vi "MainGUI.vi"(0 "reference in":refnum<class "UserManager.lvclass">, 5 "Error In":errorcluster) -> (14 "reference out":refnum<class "UserManager.lvclass">, 19 "Error Out":errorcluster)   [LabVIEW 2021]
doc: "This template is based off of the Queued Message Handler design pattern and the Queued Message Handler project template that ships with LabVIEW.\n\nThe main difference is that the queue is private to this module and communication between modules is performed via Broadcast and Request events.\n\nRequest events are wrapped in public API methods and are handled in the Event Handling Loop (EHL) of this VI. Any module can register for Broadcast events sent by this module. The EHL generates messages based on user interface actions.\n\nThe Message Handling Loop (MHL) processes messages generated by the EHL, or by other messages. The messages are string values, so new messages can be added easily to the Message Cases case structure in the MHL. Each message cluster can also provide an optional value for Message Data, which is a variant that can be converted to whatever message-specific data is required.\n_____\nBased on Delacor QMH Project Template 4.2.0.63.\n\n<b>Note:</b> This VI was modified by the <b>Validate DQMH Module</b> tool to have the module name be passed as the Additional Information parameter with an Error Reported broadcast.\n\n<b>Note:</b> This VI was modified by the <b>Validate DQMH Module</b> tool to call the Release Message Queue VI in the top-level Error case."
uses:
  .Externals/Library_TAF_UserManager/UserManager/UserManager/protected/UserManager_MessageData.ctl
  .Externals/Library_TAF_UserManager/UserManager/UserManager/UserManager.lvclass
panel:
  out "Last Command":string
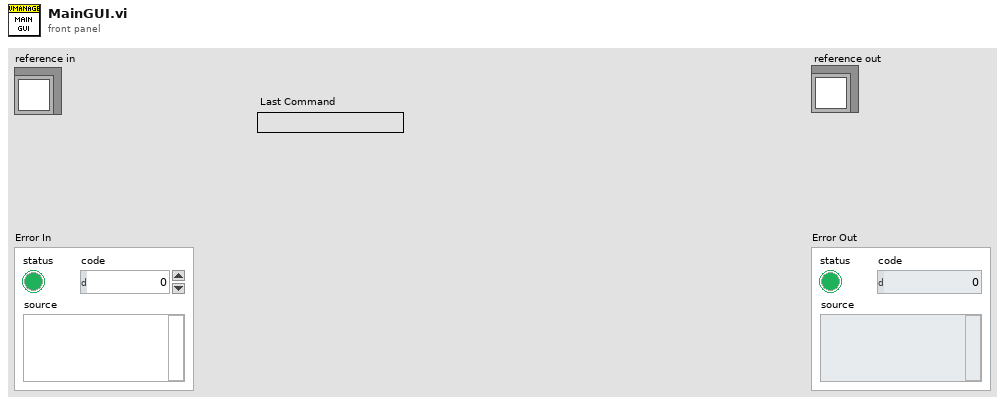
[diagram p1: front panel]
types:
  T1 = typedef "UserMananger.lvlib/UserManager.lvclass/UserManager_MessageData.ctl" = cluster{"ShowWindow":cluster{"Send":cluster{"Show":bool}, "Receive":cluster{"Dummy":bool}}}
  T2 = cluster{"Event":refnum<event-registration>, "Command":string, "MessageData":T1, "ReplyQueue":refnum<queue>}
  T3 = cluster{"ReplyQueue":refnum<queue>, "Data":variant}
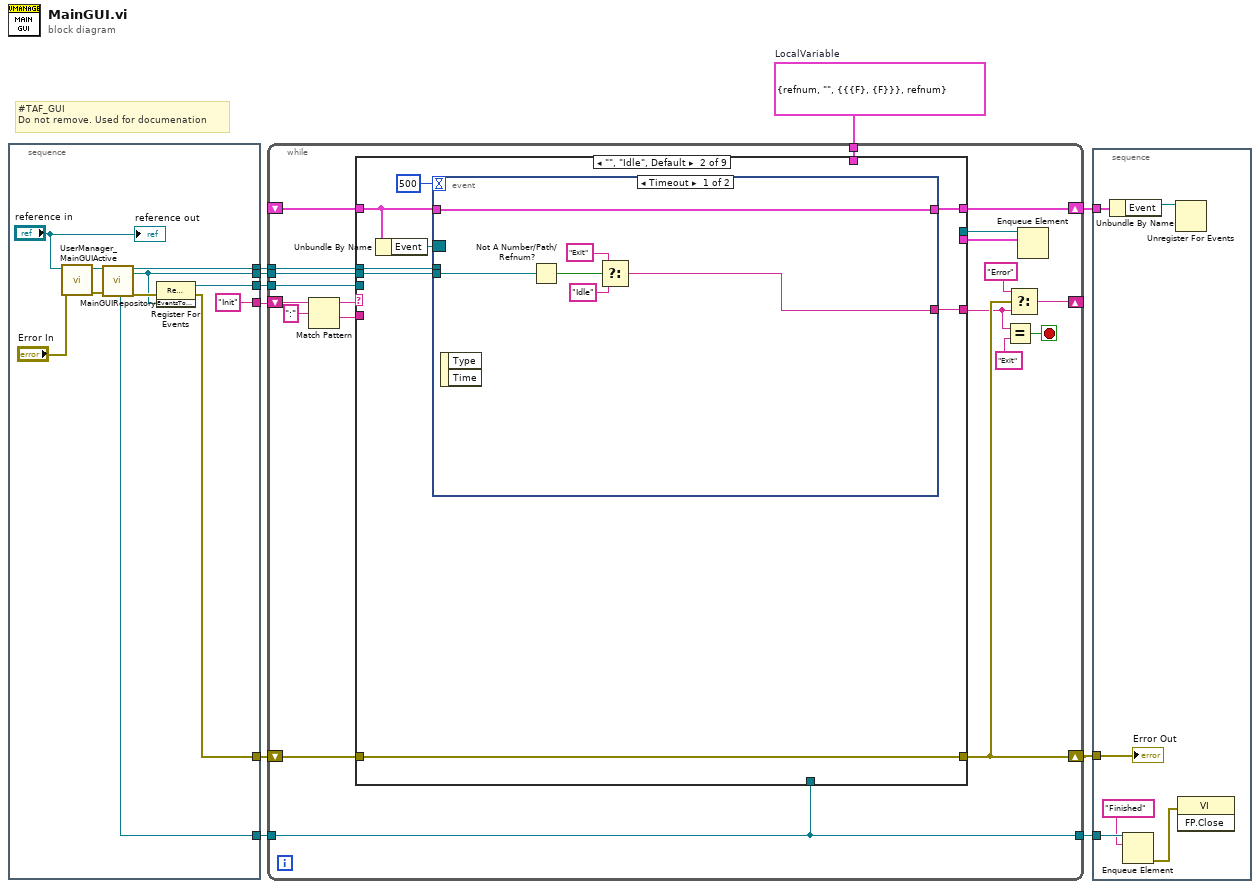
[diagram p0: block diagram]
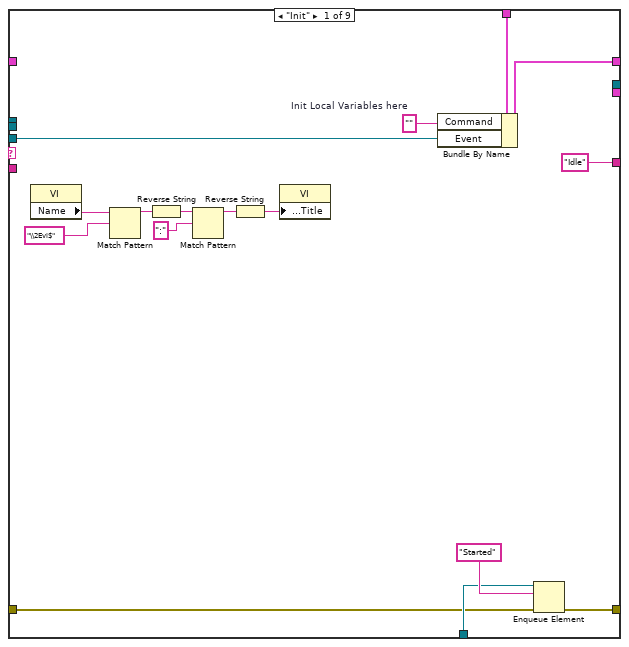
[diagram p2: hidden frame]
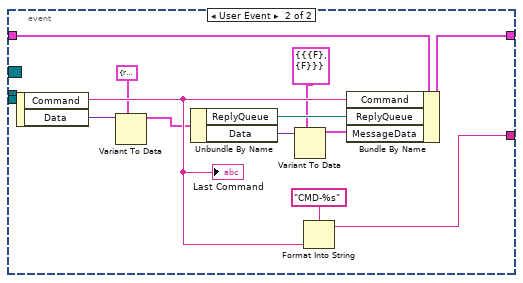
[diagram p3: hidden frame]
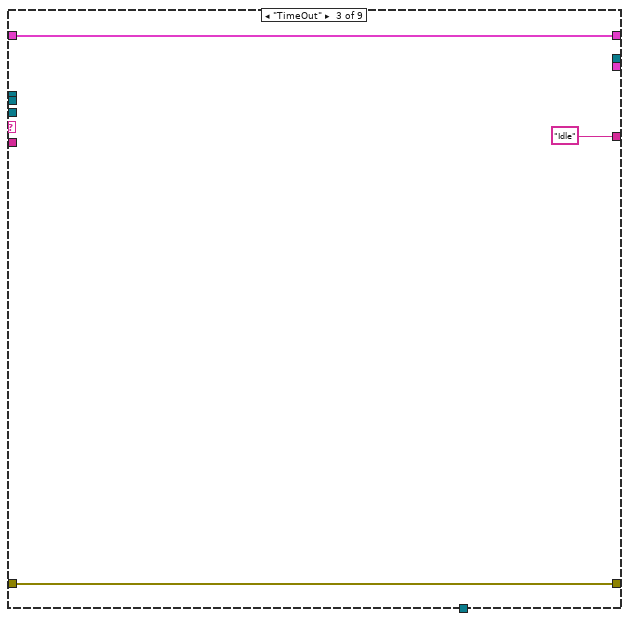
[diagram p4: hidden frame]
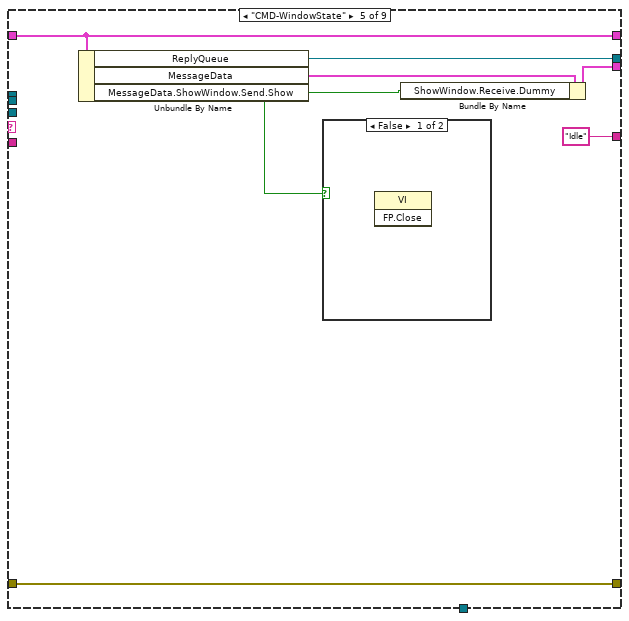
[diagram p6: hidden frame]
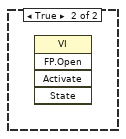
[diagram p7: hidden frame]
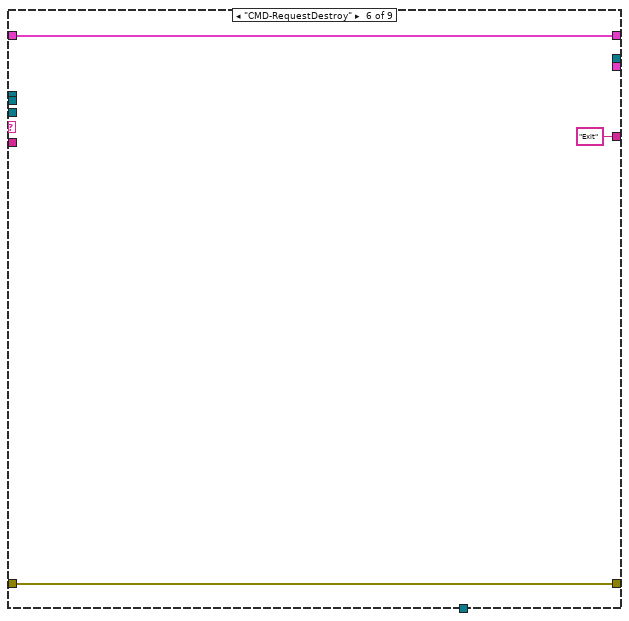
[diagram p8: hidden frame]
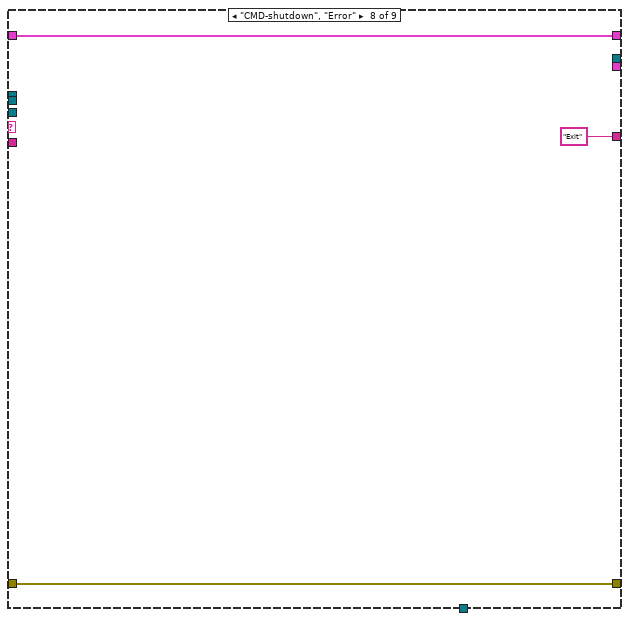
[diagram p10: hidden frame]
diagram:
  w5 = T2 {"Event"=refnum, "Command"="", "MessageData"={"ShowWindow"={"Send"={"Show"=FALSE}, "Receive"={"Dummy"=FALSE}}}, "ReplyQueue"=refnum}  # LocalVariable
  # "#TAF_GUI\nDo not remove. Used for documenation"
  n1 = stacked-sequence {
    tunnel: [w15] -> w10
    tunnel: [w21] -> w8
    tunnel: [w18] -> w7
    tunnel: ["Init"] -> w6
    tunnel: [w16] -> w3
    tunnel: [w11] -> w1
    frame #0 {
      n2 = call "UserManager_MainGUIActive.vi"("ErrorIn"="Error In", "ReferenceIn"="reference in") -> ("ErrorOut"=w12:errorcluster, "ReferenceOut"=w14:refnum<class "UserManager.lvclass">)  [unwired: 8 in]
      n3 = call "MainGUIRepository.vi"("ReferenceIn"=w14, "ErrorIn"=w12) -> ("ProcessSyncQueue"=w16:refnum<queue>, "ReferenceOut"=w21:refnum<class "UserManager.lvclass">, "EventsToProcess"=w11:refnum<user-event>, "ErrorOut"=w17:errorcluster)  [unwired: 10 in, 4 out]
      n4 = register-events(error in=w17, w11) -> (reference out=w18:refnum<event-registration>, error out=w15:errorcluster)  [unwired: 1 in]
      "reference out" <- "reference in"
    }
  }
  n5 = while {
    shift-right: [w34] -> w9
    shift-left: w10 -> [w39]
    tunnel: w8 -> [w40]
    tunnel: w7 -> [w41]
    shift-right: [w32] -> _
    shift-left: w6 -> [w37]
    shift-right: [w28] -> w4
    shift-left: _ -> [w27]
    tunnel: w5 -> [w26]
    tunnel: [w23] -> w2
    tunnel: w3 -> [w23]
    tunnel: w1 -> [w22]
    stop <- w29 stop-if-true
    n6 = Match Pattern(string=w37, regular expression=":") -> (before substring=w36:string, after substring=w35:string)  [unwired: 1 in, 2 out]
    n7 = case shown="\"\", \"Idle\", Default" w36 {
      tunnel: w39 -> [w42 w60 w86 w88 w95 w98 w100 w103 w105]
      tunnel: [w44 w60 w86 w88 w95 w98 w100 w103 w105] -> w34
      tunnel: w41 -> [w46 _ _ _ _ _ _ _ _]
      tunnel: w40 -> [_ w59 _ _ _ _ _ _ _]
      tunnel: w35 -> [_ _ _ _ _ _ _ _ _]
      tunnel: ["Idle" ("t") w65 "Idle" ("t") _ "Idle" ("t") "Exit" ("y") _ "Exit" ("y") _] -> w31
      tunnel: [w57 w64 w84 w87 w93 w97 w99 w101 w104] -> w28
      tunnel: w27 -> [_ w63 w84 w87 w93 w97 w99 w101 w104]
      tunnel: w26 -> [w54 _ _ _ _ _ _ _ _]
      tunnel: [_ _ _ _ w92 _ _ _ _] -> w25
      tunnel: [_ _ _ _ w90 _ _ _ _] -> w24
      tunnel: w23 -> [w43 _ _ _ _ _ _ _ _]
      tunnel: w22 -> [_ w58 _ _ _ _ _ _ _]
      frame "Init" {
        w56 = ""  # Init Local Variables here
        n8 = property class="VI"() -> ("Name"=w53:string)  [unwired: 2 in, 2 out]
        n9 = Match Pattern(string=w53, regular expression="\\2Evi$") -> (before substring=w51:string)  [unwired: 1 in, 3 out]
        n10 = Reverse String(1:w51) -> (0:w50:string)
        n11 = Match Pattern(string=w50, regular expression=":") -> (before substring=w48:string)  [unwired: 1 in, 3 out]
        n12 = Reverse String(1:w48) -> (0:w47:string)
        n13 = property class="VI"("Front Panel.Title"=w47) -> ()  [unwired: 2 in, 2 out]
        n14 = Bundle By Name(cluster=w54, "Command"=w56, "Event"=w46) -> (w57:T2)
        n15 = Enqueue Element(queue=w43, element="Started", error in (no error)=w42) -> (error out=w44:errorcluster)  [unwired: 1 in, 2 out]
      }
      frame "", "Idle", Default {
        n16 = Unbundle By Name(w63) -> ("Event"=w62:refnum<event-registration>)
        n17 = event shown="[0] Timeout" {
          selector: w62 -> [_ _]
          dyn-events: _ -> [_ _]
          timeout: 500 -> [_ _]
          tunnel: [w66 w80] -> w65
          tunnel: w63 -> [w71 w83]
          tunnel: [w71 w82] -> w64
          tunnel: w59 -> [_ _]
          tunnel: w58 -> [w67 _]
          event Timeout {
            n18 = event-data() -> ()  [unwired: 1 in, 2 out]
            n19 = Not A Number/Path/Refnum?(number/path/refnum=w67) -> (NaN/Path/Refnum?=w68:bool)
            n20 = Select(t="Exit", s=w68, f="Idle" ("t")) -> (s? t:f=w66:string)
          }
          event User Event {
            n21 = event-data() -> ("Command"=w79:string, "Data"=w78:variant)  [unwired: 1 in]
            "Last Command" <- w79
            n22 = Variant To Data(type=T3 {"ReplyQueue"=refnum, "Data"=variant} ("output cluster"), Variant=w78) -> (data=w76:T3)  [unwired: 1 in, 1 out]
            n23 = Unbundle By Name(w76) -> ("ReplyQueue"=w75:refnum<queue>, "Data"=w74:variant)
            n24 = Variant To Data(type=T1 {"ShowWindow"={"Send"={"Show"=FALSE}, "Receive"={"Dummy"=FALSE}}} ("MessageData"), Variant=w74) -> (data=w73:T1)  [unwired: 1 in, 1 out]
            n25 = Format Into String(format string="CMD-%s", w79) -> (resulting string=w80:string)  [unwired: 2 in, 1 out]
            n26 = Bundle By Name(cluster=w83, "Command"=w79, "ReplyQueue"=w75, "MessageData"=w73) -> (w82:T2)
          }
        }
      }
      frame "TimeOut" {
      }
      frame "---- COMMANDS START----" {
      }
      frame "CMD-WindowState" {
        n27 = Unbundle By Name(w93) -> ("ReplyQueue"=w92:refnum<queue>, "MessageData"=w91:T1, "MessageData.ShowWindow.Send.Show"=w89:bool)
        n28 = case shown="False" w89 {
          frame False {
            n29 = invoke class="VI" method="FP.Close"() -> ()  [unwired: 3 in, 3 out]
          }
          frame True {
            n30 = invoke class="VI" method="FP.Open"() -> ()  [unwired: 5 in, 5 out]
          }
        }
        n31 = Bundle By Name(cluster=w91, "ShowWindow.Receive.Dummy"=w89) -> (w90:T1)
      }
      frame "CMD-RequestDestroy" {
      }
      frame "----- COMMANDS END ----" {
      }
      frame "CMD-shutdown", "Error" {
      }
      frame "----- UI ACTIONS -----" {
      }
    }
    n32 = Equal?(x=w31, y="Exit") -> (x = y?=w29:bool)
    n33 = Select(t="Error", s=w34, f=w31) -> (s? t:f=w32:string)
    n34 = Enqueue Element(queue=w25, element=w24) -> ()  [unwired: 2 in, 3 out]
  }
  n35 = stacked-sequence {
    tunnel: w9 -> [w111]
    tunnel: w2 -> [w108]
    tunnel: w4 -> [w110]
    frame #0 {
      n36 = Unbundle By Name(w110) -> ("Event"=w109:refnum<event-registration>)
      n37 = Enqueue Element(queue=w108, element="Finished") -> (error out=w107:errorcluster)  [unwired: 2 in, 2 out]
      n38 = Unregister For Events(event registration refnum=w109) -> ()  [unwired: 1 in, 1 out]
      n39 = invoke class="VI" method="FP.Close"(error in=w107) -> ()  [unwired: 2 in, 3 out]
      "Error Out" <- w111
    }
  }
